vi "GEA2 Scale ERD Data.vi"(0 "HEWH ERD Data":T2 {"ERD Therm Data"."EEV Possition" format="%0.0f"; "ERD Therm Data"."T6" format="%.1f"; "ERD Therm Data"."T2" format="%.1f"; "ERD Therm Data"."T3a" format="%.1f"; "ERD Therm Data"."T3b" format="%.1f"; "ERD Therm Data"."T4" format="%.1f"; "ERD Therm Data"."T5" format="%.1f"; "ERD Therm Data"."Current" format="%.1f"}, 3 "Raw Data":string[](array[string]), 5 "ERD_Data_Bundled_Out":T5, 9 "Headers":string[](array[string]), 11 "Error In":errorcluster, 12 "LV Program":T1, 13 "Disable Electronic Mixing Valve (EMV) List":bool, 14 "Disable ERD (Main)":bool) -> (4 "ERD Array":string[][](array[string]), 15 "Error Out":errorcluster)   [LabVIEW 2016]
uses:
  type defs/HEWH ERD Data.ctl
  type defs/HEWH Faults.ctl
  type defs/HEWH Mixing Valve.ctl
  type defs/ERD_Data_Bundled.ctl
  Washer HCC/Washer HCC NEWFI/Washer Soft Load Box/type defs/ATC_Data.ctl
  Washer HCC/Washer HCC NEWFI/Washer Soft Load Box/type defs/Redundant.ctl
  Washer HCC/Washer HCC NEWFI/Washer Soft Load Box/type defs/Version.ctl
  Washer HCC/Washer HCC NEWFI/Washer Soft Load Box/type defs/Algorithms.ctl
  Washer HCC/Washer HCC NEWFI/Washer Soft Load Box/type defs/ERD_Always_Show.ctl
  Washer HCC/Washer HCC NEWFI/Washer Soft Load Box/type defs/Fault_Table_Info.ctl
  Save File/File Setup (Public)/Type Definition/Save File DOE LabView Program.ctl
  <vilib>/Utility/error.llb/whitespace.ctl
  Save File/File Setup.lvlib
panel:
  in  "Tab Control":enum32{"HEWH", "Washer"}(tab)
  # "Wet Load Size"
  # "Dry Load Size"
  # "OOB"
  # "Software Version"
  # "Critical Version"
  # "Non-Critical"
  # "XML Crit Ver"
  # "XML Non-Crit"
  # "Daily Build"
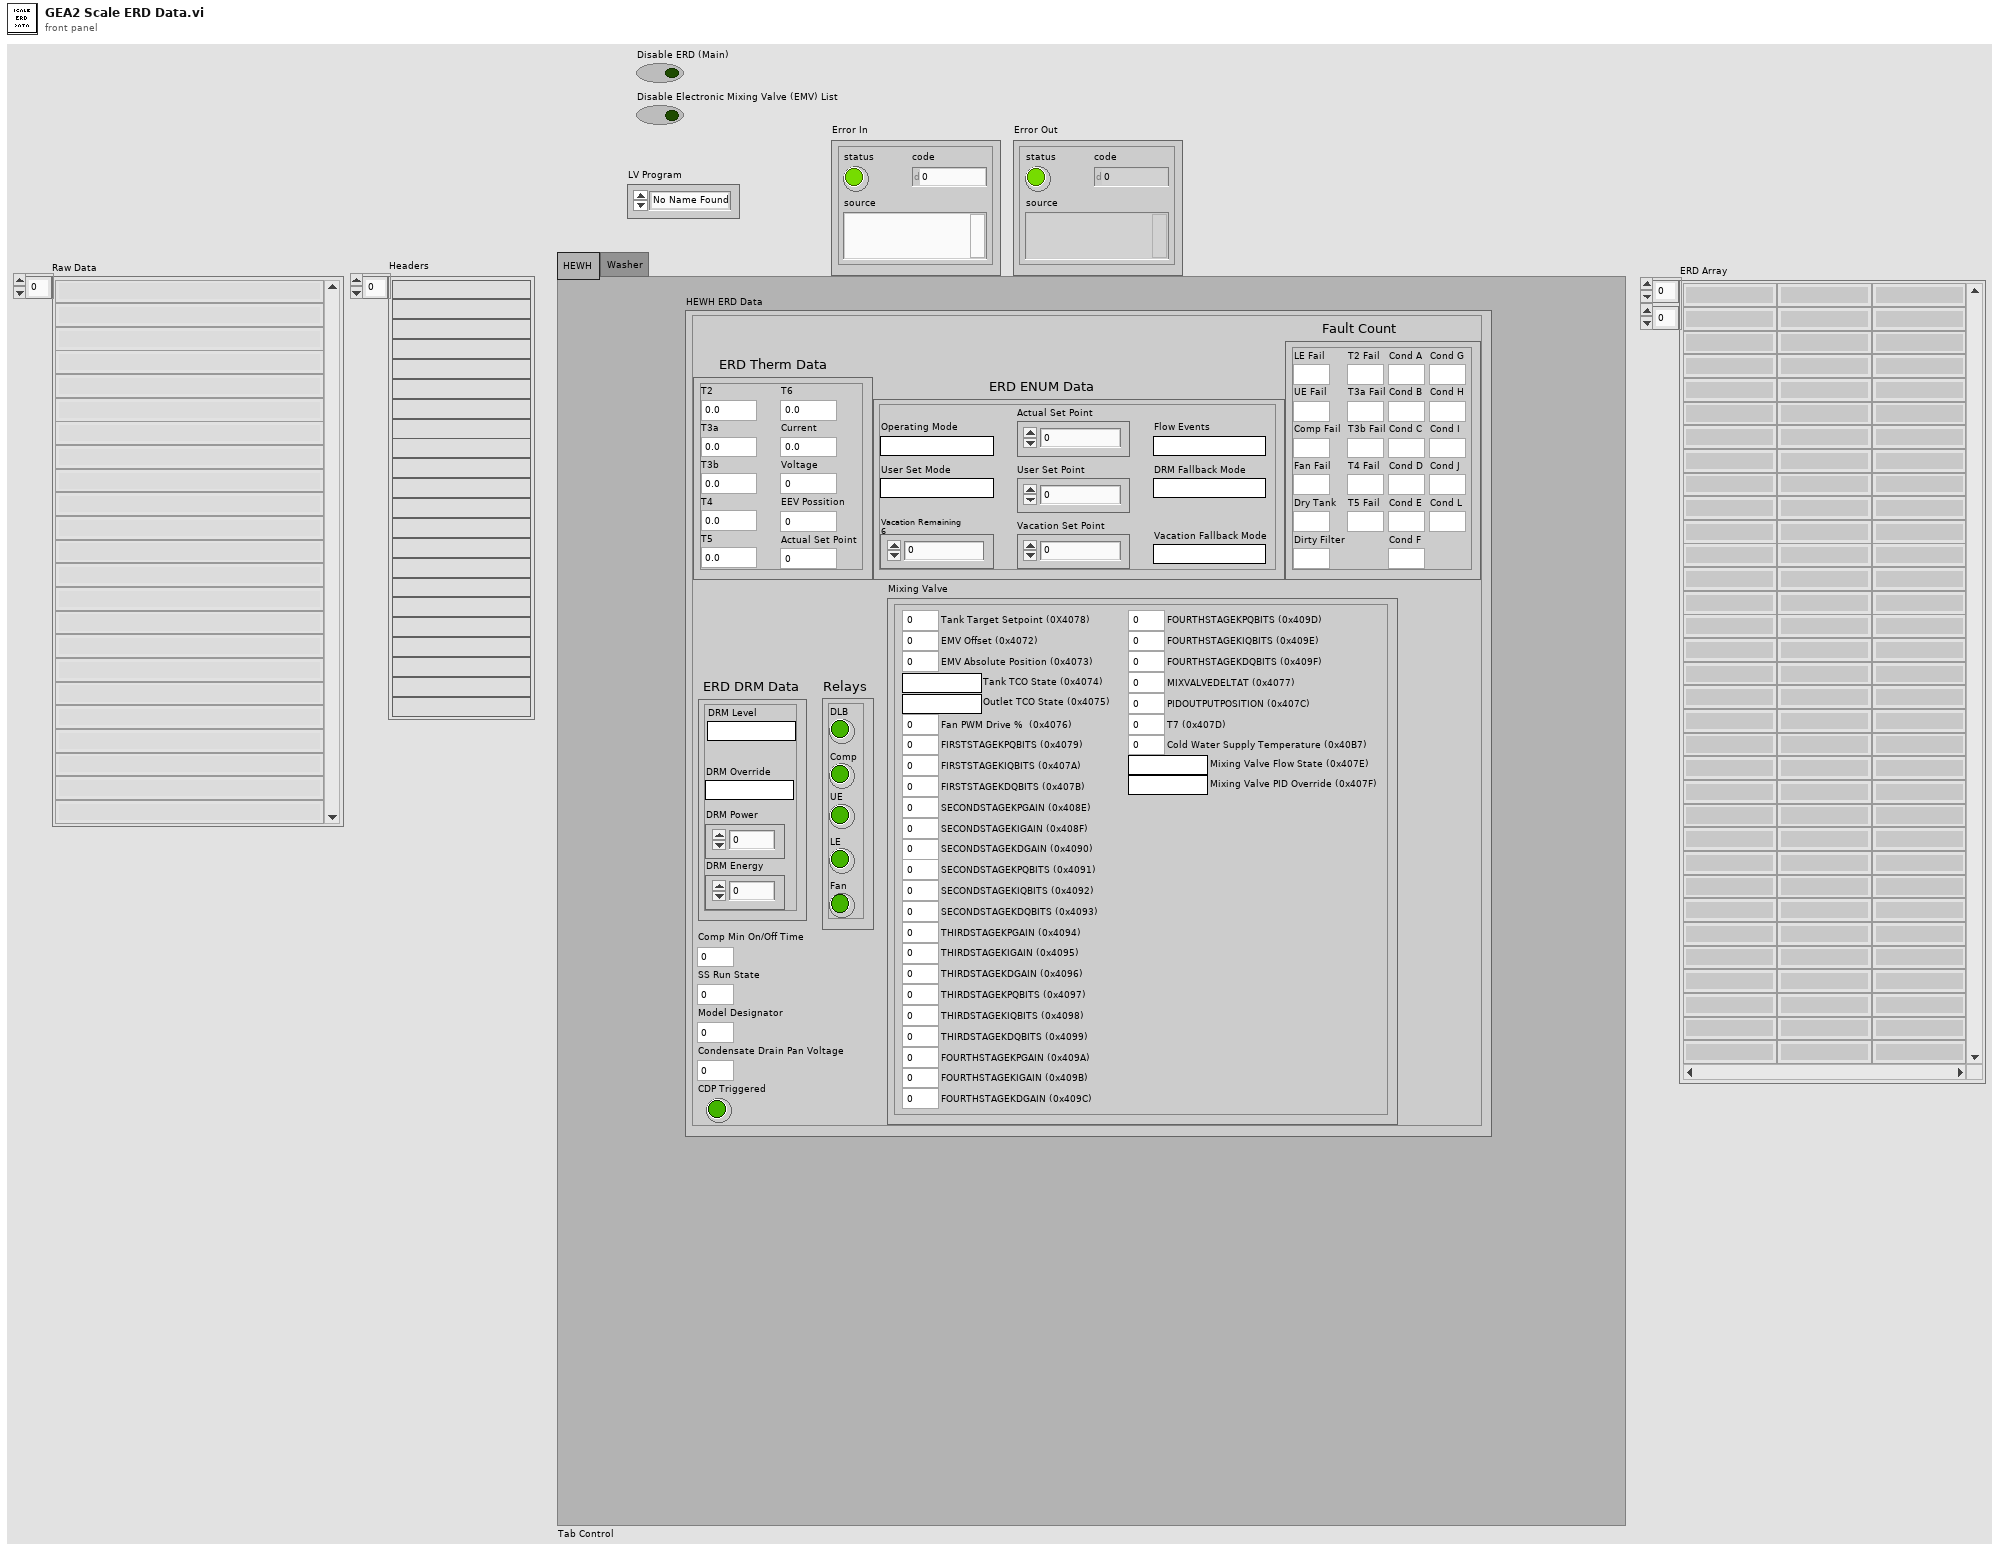
[diagram p1: front panel]
types:
  T1 = typedef "File Setup.lvlib/Save File DOE LabView Program.ctl" = enum16{"No Name Found", "DOE Stand", "Dishwasher Kitchen", "Portable Stand", "HEWH", "Dryer", "Dryer WILT", "HCC", "PRAT", "HEWH RLT", "Refrigeration"}
  T2 = typedef "HEWH ERD Data.ctl" = cluster{"ERD Therm Data":cluster{"T2":dbl, "T3a":dbl, "T3b":dbl, "T4":dbl, "T5":dbl, "T6":dbl, "Current":dbl, "Voltage":dbl, "EEV Possition":dbl, "Actual Set Point":dbl}, "ERD ENUM Data":cluster{"Actual Set Point":dbl, "Flow Events":string, "User Set Mode":string, "Operating Mode":string, "DRM Fallback Mode":string, "Vacation Fallback Mode":string, "User Set Point":dbl, "Vacation Set Point":dbl, "Vacation Remaining\n6":dbl}, "ERD DRM Data":cluster{"DRM Level":string, "DRM Override":string, "DRM Power":dbl, "DRM Energy":dbl}, "Fault Count":T3, "Relays":cluster{"DLB":bool, "Comp":bool, "UE":bool, "LE":bool, "Fan":bool}, "Comp Min On/Off Time":u16, "SS Run State":u16, "Condensate Drain Pan Voltage":u16, "CDP Triggered":bool, "Model Designator":u8, "Mixing Valve":T4}
  T3 = typedef "HEWH Faults.ctl" = cluster{"LE Fail":u32, "UE Fail":u32, "Comp Fail":u32, "T2 Fail":u32, "T3a Fail":u32, "T3b Fail":u32, "T4 Fail":u32, "T5 Fail":u32, "Cond A":u32, "Cond B":u32, "Cond C":u32, "Cond D":u32, "Cond E":u32, "Cond F":u32, "Cond G":u32, "Cond H":u32, "Cond I":u32, "Cond J":u32, "Cond L":u32, "Fan Fail":u32, "Dirty Filter":u32, "Dry Tank":u32}
  T4 = typedef "HEWH Mixing Valve.ctl" = cluster{"Tank Target Setpoint (0X4078)":dbl, "EMV Offset (0x4072)":dbl, "EMV Absolute Position (0x4073)":dbl, "Tank TCO State (0x4074)":string, "Outlet TCO State (0x4075)":string, "Fan PWM Drive %  (0x4076)":dbl, "FIRSTSTAGEKPQBITS (0x4079)":dbl, "FIRSTSTAGEKIQBITS (0x407A)":dbl, "FIRSTSTAGEKDQBITS (0x407B)":dbl, "SECONDSTAGEKPGAIN (0x408E)":dbl, "SECONDSTAGEKIGAIN (0x408F)":dbl, "SECONDSTAGEKDGAIN (0x4090)":dbl, "SECONDSTAGEKPQBITS (0x4091)":dbl, "SECONDSTAGEKIQBITS (0x4092)":dbl, "SECONDSTAGEKDQBITS (0x4093)":dbl, "THIRDSTAGEKPGAIN (0x4094)":dbl, "THIRDSTAGEKIGAIN (0x4095)":dbl, "THIRDSTAGEKDGAIN (0x4096)":dbl, "THIRDSTAGEKPQBITS (0x4097)":dbl, "THIRDSTAGEKIQBITS (0x4098)":dbl, "THIRDSTAGEKDQBITS (0x4099)":dbl, "FOURTHSTAGEKPGAIN (0x409A)":dbl, "FOURTHSTAGEKIGAIN (0x409B)":dbl, "FOURTHSTAGEKDGAIN (0x409C)":dbl, "FOURTHSTAGEKPQBITS (0x409D)":dbl, "FOURTHSTAGEKIQBITS (0x409E)":dbl, "FOURTHSTAGEKDQBITS (0x409F)":dbl, "MIXVALVEDELTAT (0x4077)":dbl, "PIDOUTPUTPOSITION (0x407C)":dbl, "T7 (0x407D)":dbl, "Cold Water Supply Temperature (0x40B7)":dbl, "Mixing Valve Flow State (0x407E)":string, "Mixing Valve PID Override (0x407F)":string}
  T5 = typedef "ERD_Data_Bundled.ctl" = cluster{"ATC Data":T6, "Redundant Micro":T7, "Version":T8, "Algorithm Data":T9, "ERD_Always Show":T10, "ERD Graph  Ind":cluster{"ERD Value 1":dbl, "ERD Value 2":dbl, "ERD Value 3":dbl}, "Personality Set":u8, "Fault Table Entry":T11[]}
  T6 = typedef "ATC_Data.ctl" = cluster{"Current Tub Gallons":dbl, "Hot Gallons":dbl, "Cold Gallons":dbl, "Target Gallons":dbl, "Current Water Temp":dbl, "Target Level":u32, "Target Bath Temp":dbl, "Current Bath Temp ":dbl, "Cold Inlet Temp":dbl, "Hot Inlet Temp":dbl, "Warm Inlet Temp":dbl, "Hot Seg Valve Time":u16, "Cold Seg Valve Time ":u16, "User Temp Level":string, "Segment Gallons":dbl}
  T7 = typedef "Redundant.ctl" = cluster{"Version":string, "Personality":u8, "Pressure ":dbl, "Shaft Speed":u16, "Modeshift Feedback":string, "Lid Switch":bool, "Lid Lock":bool, "Triac Enable":bool, "Drain Pump":bool, "Lid Lock Motor Speed Safety Interlock":bool, "Flood Condition State":bool, "Lid Open Fault State":bool, "Access To Moving Parts State":bool, "Heartbeat":bool, "Motor Enable":bool, "Lid Unlock Fault State":bool}
  T8 = typedef "Version.ctl" = cluster{"Critical Major":string, "Critical Minor":string, "Non-Critical Minor":string, "Non-Critical Major":string, "XML Crit Minor":string, "XMLCrit Major":string, "Daily Rev":string, "XML Non-crit Minor":string, "Xml Non-crit Major":string}
  T9 = typedef "Algorithms.ctl" = cluster{"Wet Load Gal":dbl, "Target Gallons":dbl, "Load Type":string, "Load Size":string, "Coast Time":u16, "Ramp Time":u16, "Ramp  Speed":u16, "Ramp Avg Current":dbl, "OOB Redist Req":bool, "OOB Detected in S-S":bool, "Max Accel in Accel":i32, "Max Jerk in Accel":i32, "Max Jerk in S-S":i32, "OOB Detected in Accel":bool, "Partial Coast Time":u16, "Dry Load Size":dbl, "Ramp Line Voltage ":dbl, "Coast Line Voltage":dbl}
  T10 = typedef "ERD_Always_Show.ctl" = cluster{"Basket Speed (RPM)":u16, "Machine State":string, "Tub Volume (Gal)":dbl, "Pressure (inches H20)":dbl, "Lid Switch ":bool, "Current RMS (Amps)":dbl, "Cycle Selected":string, "Lid Lock Status":string, "Mode Shift Status":string, "Spray/Rinse Valve":bool, "Fabric Soft Valve":bool, "Drain Pump":bool, "Recirc. Pump":bool, "Cycle Engine State":string, "Hot  Water Valve":bool, "Cold Water Valve":bool, "Motor Profile":string, "Motor Profile Status":string, "Motor Mode":string, "ME Relay":bool, "Cycle Count":u32, "Deep Rinse / FS":bool, "My Cycle":bool, "Soil Level":string, "Spin Level":string, "Stain":string, "Temp Level":string, "Load Size":string, "Delay Time":u16, "Soak Time":u16, "Deep Fill":bool, "Warm Rinse":bool, "Auto Soak Level":string, "Extra Rinse":bool, "Wet Load Gallons":dbl, "Target Gallons":dbl, "Sub-Cycle":string, "Load Type":string, "Target Level (inches)":u32, "Valve Relay":bool, "Dry Load Size":dbl, "Shaft Speed (RPM) ":u16, "MS Motor":bool, "Mode Shift FB":bool, "Target Bath Temp (F)":dbl, "Temperature (F)":dbl, "Current Bath Temp (F)":dbl, "Lid Lock FB":string, "Lid Lock Req State":string, "Remaining Cycle Time (s)":dbl, "Available Free Stack %":u8, "Child Safety":bool, "Target Speed (RPM)":u16, "Reset Source":string}
  T11 = typedef "Fault_Table_Info.ctl" = cluster{"Cycle Count":u32, " Runtime (min) ":u32, "Fault Status":string, "Fault ID":string, "Fault Count":u16}
  T12 = typedef "whitespace.ctl" = u16
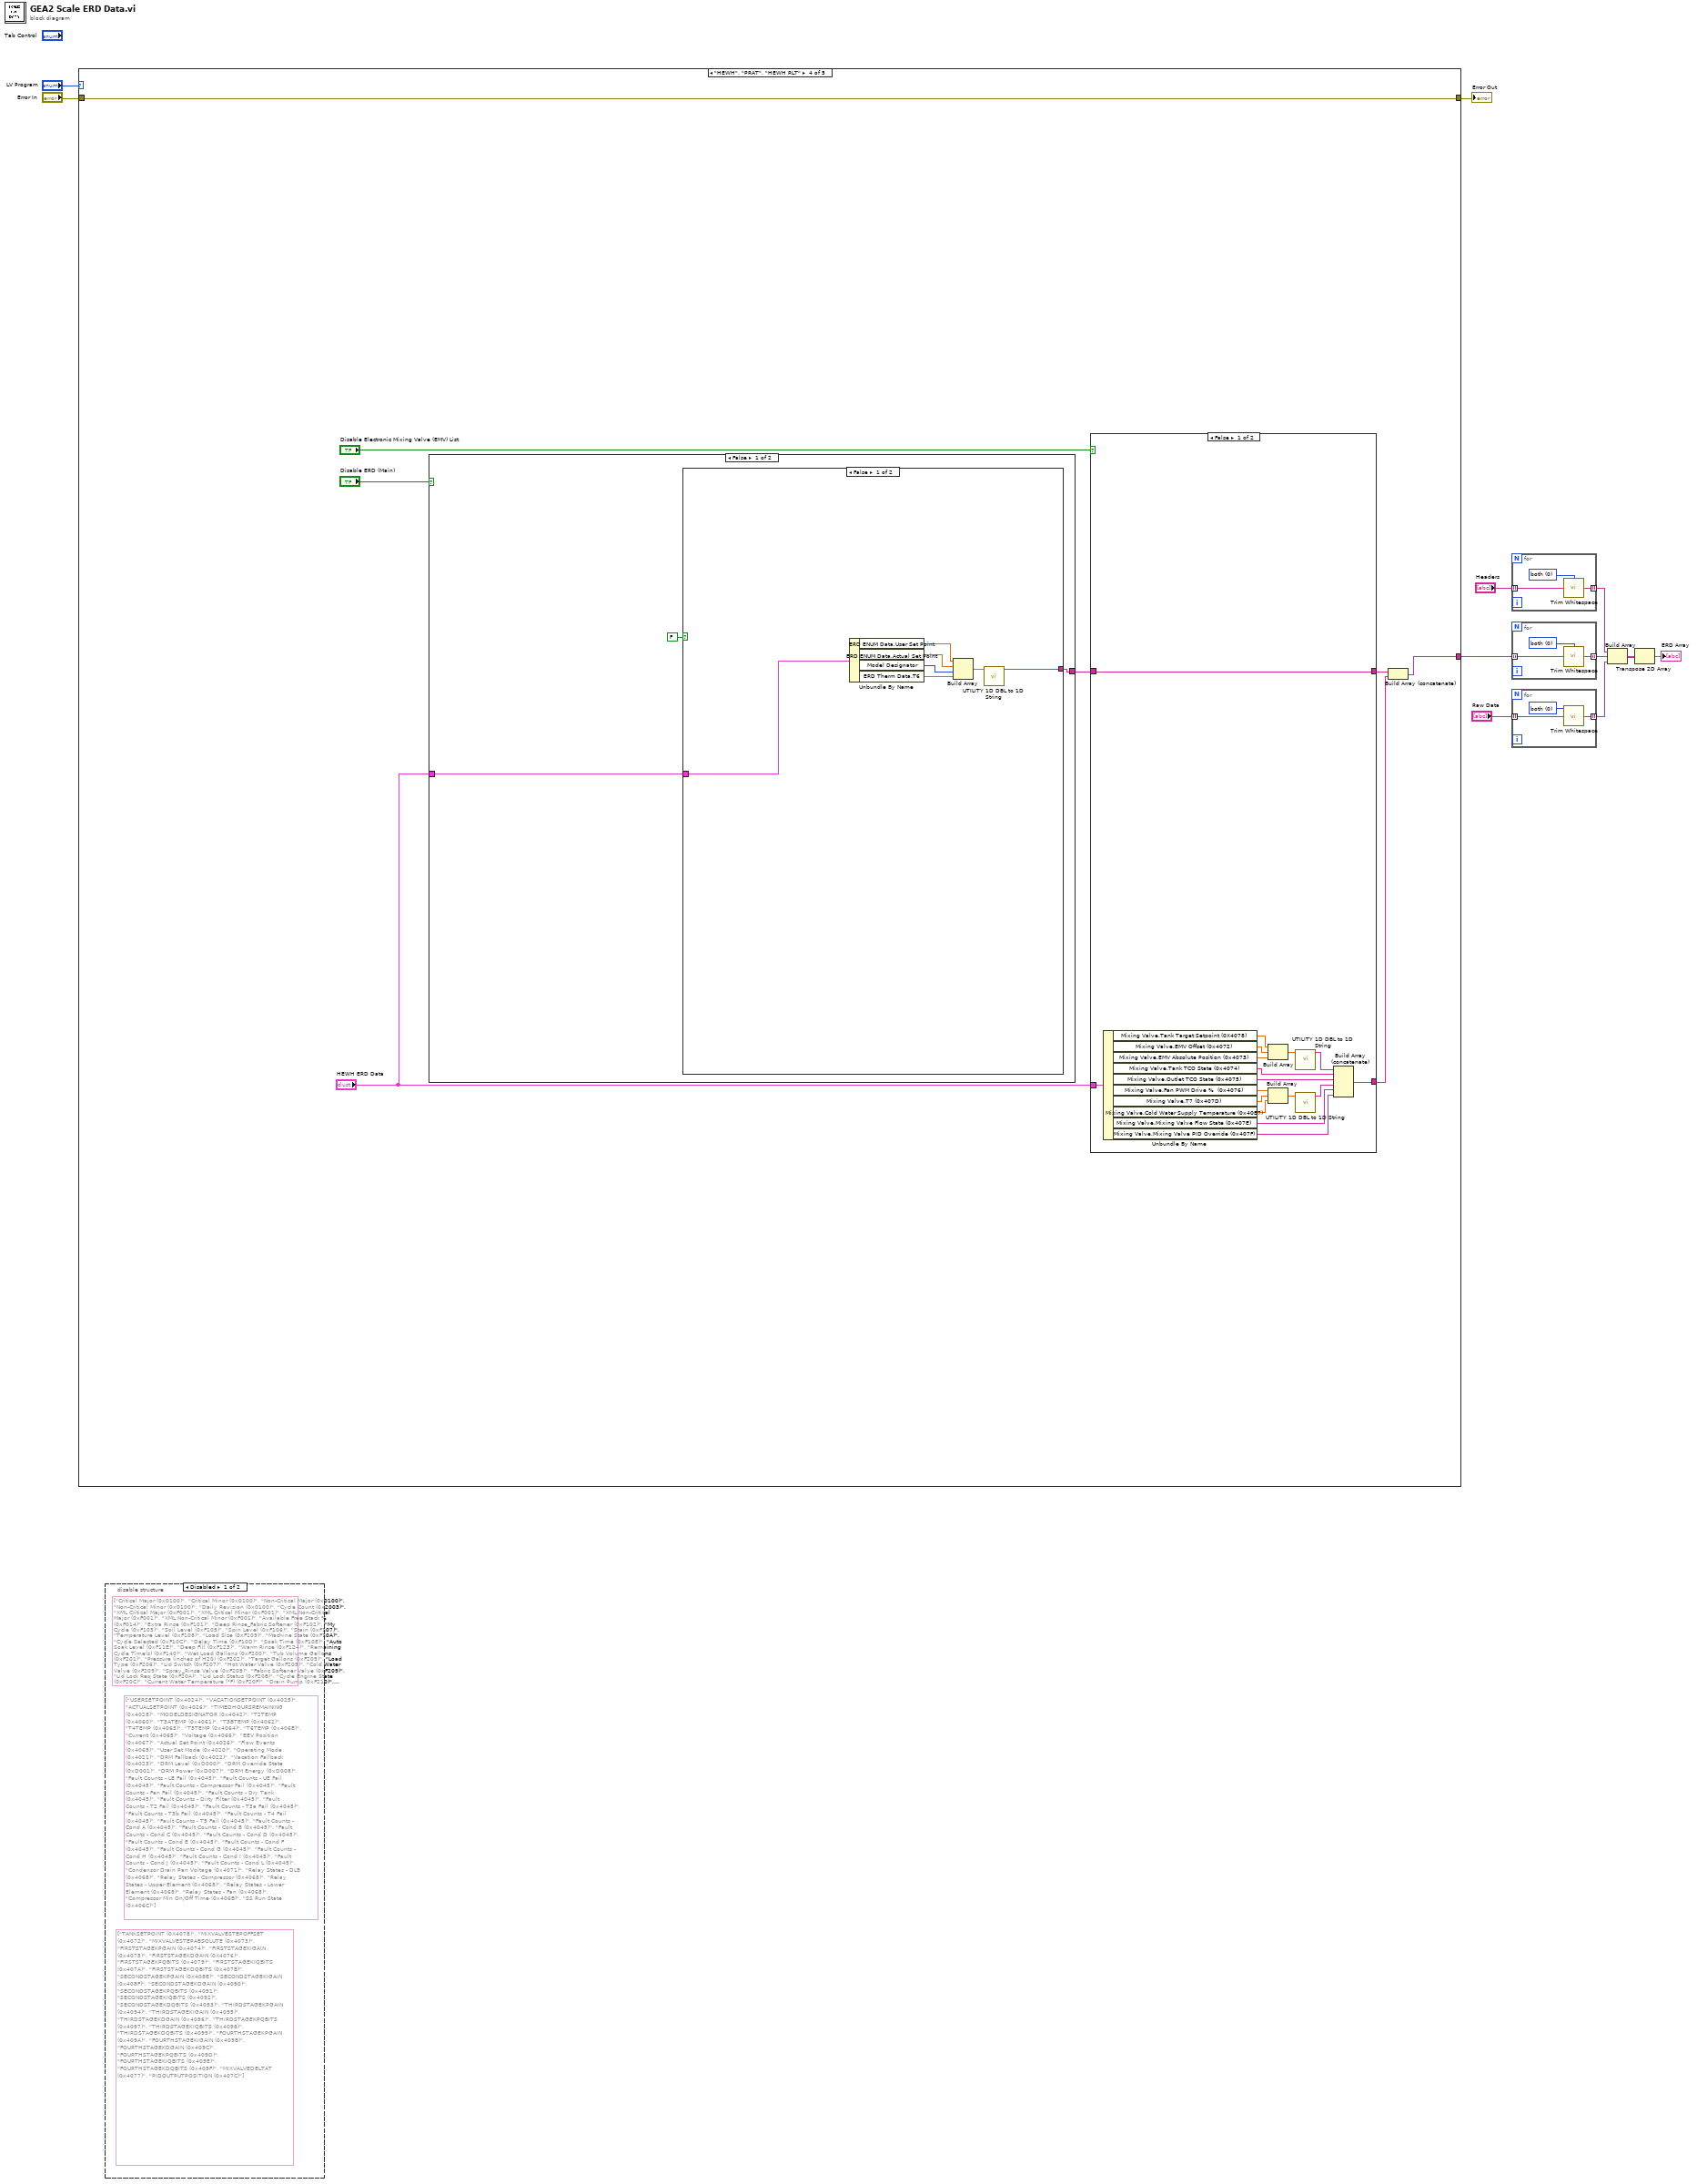
[diagram p0: block diagram]
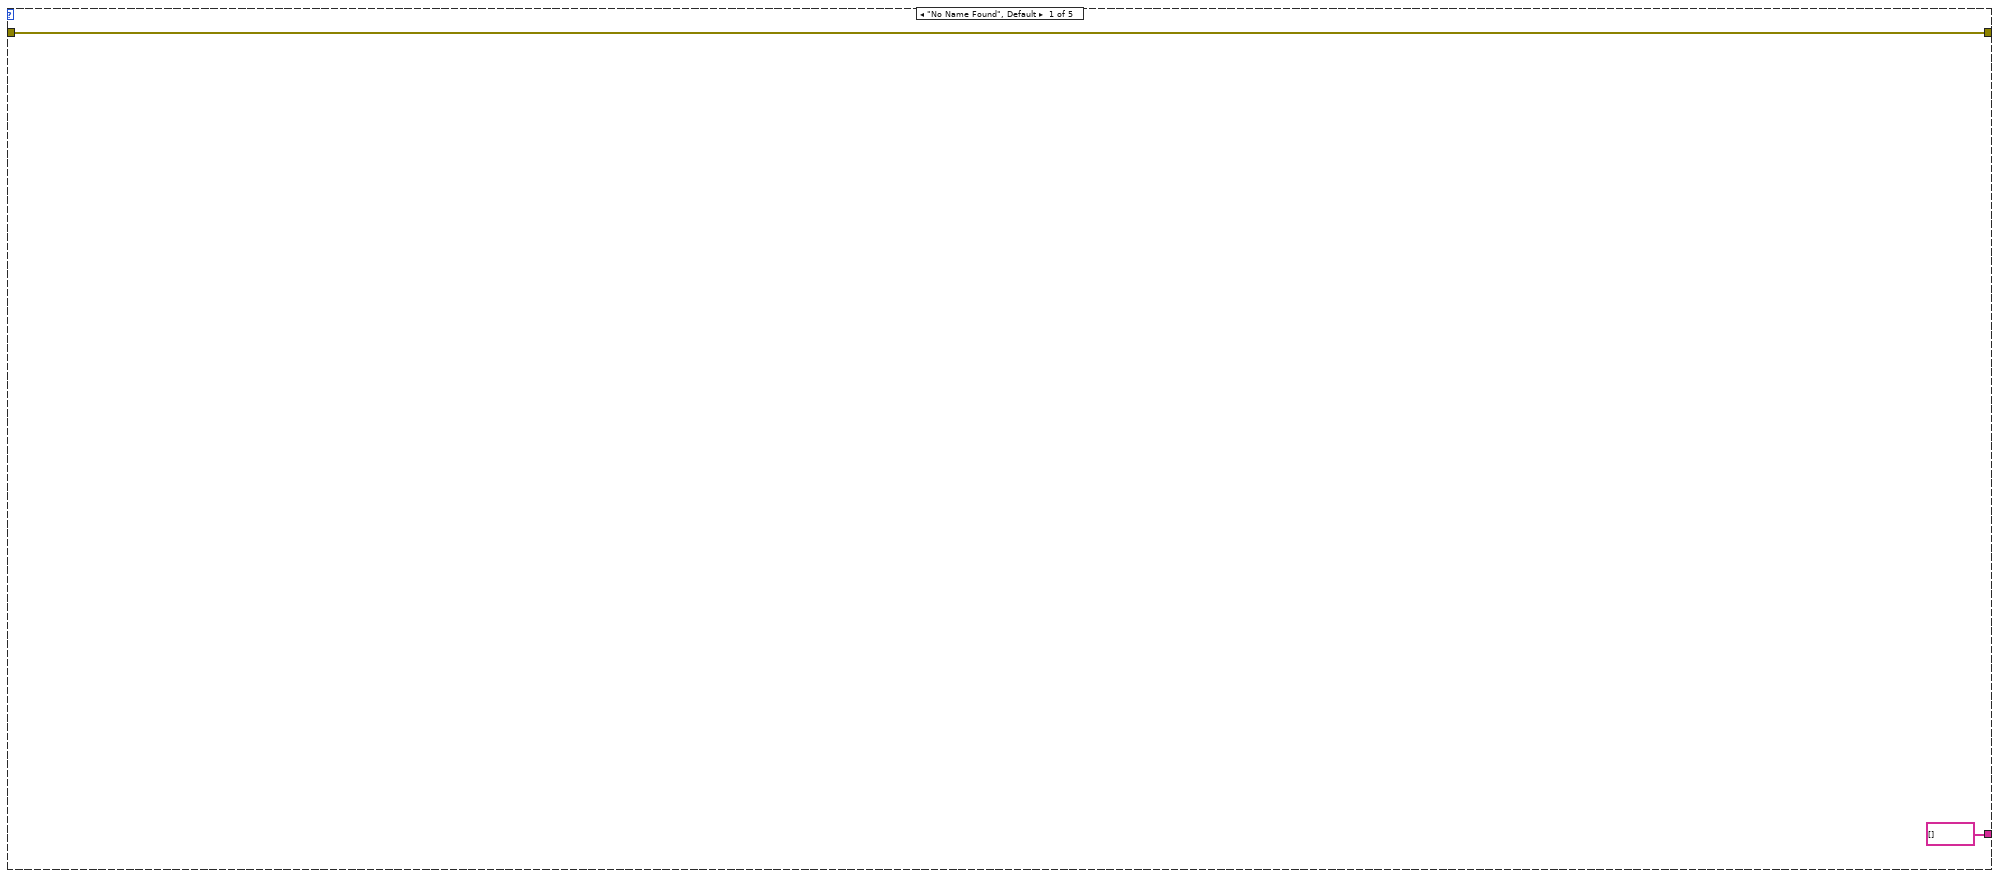
[diagram p3: hidden frame]
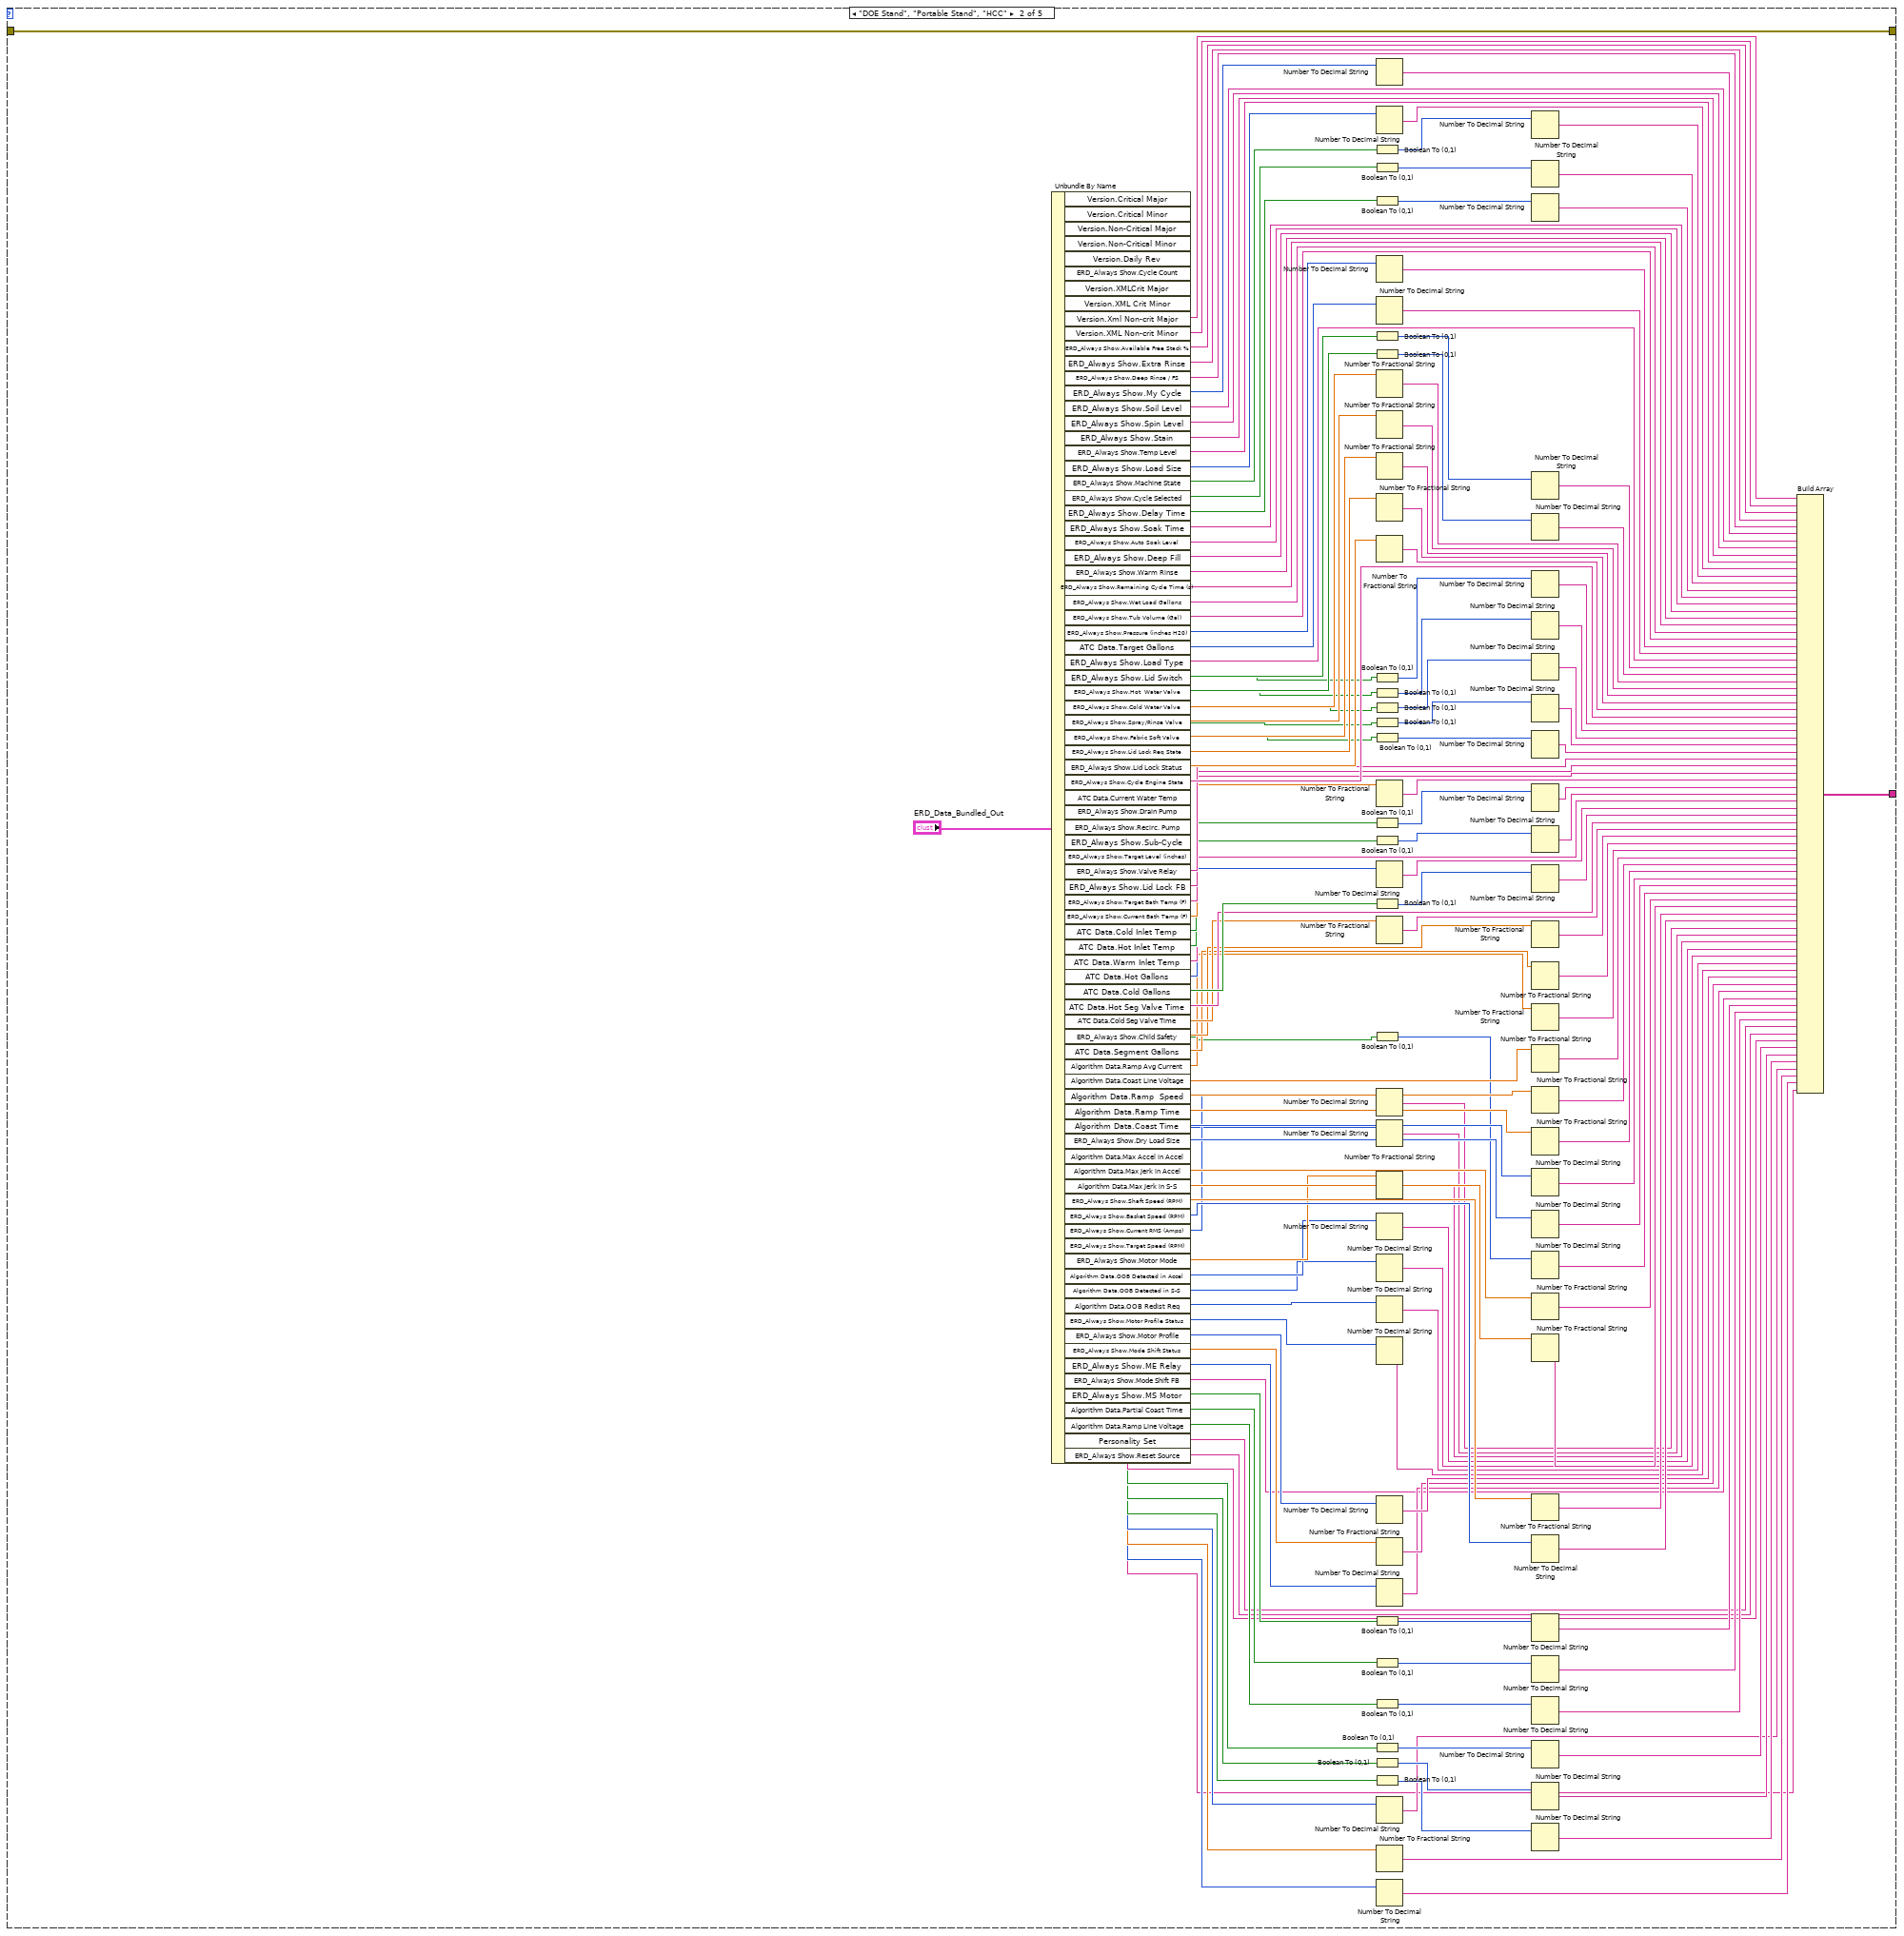
[diagram p4: hidden frame]
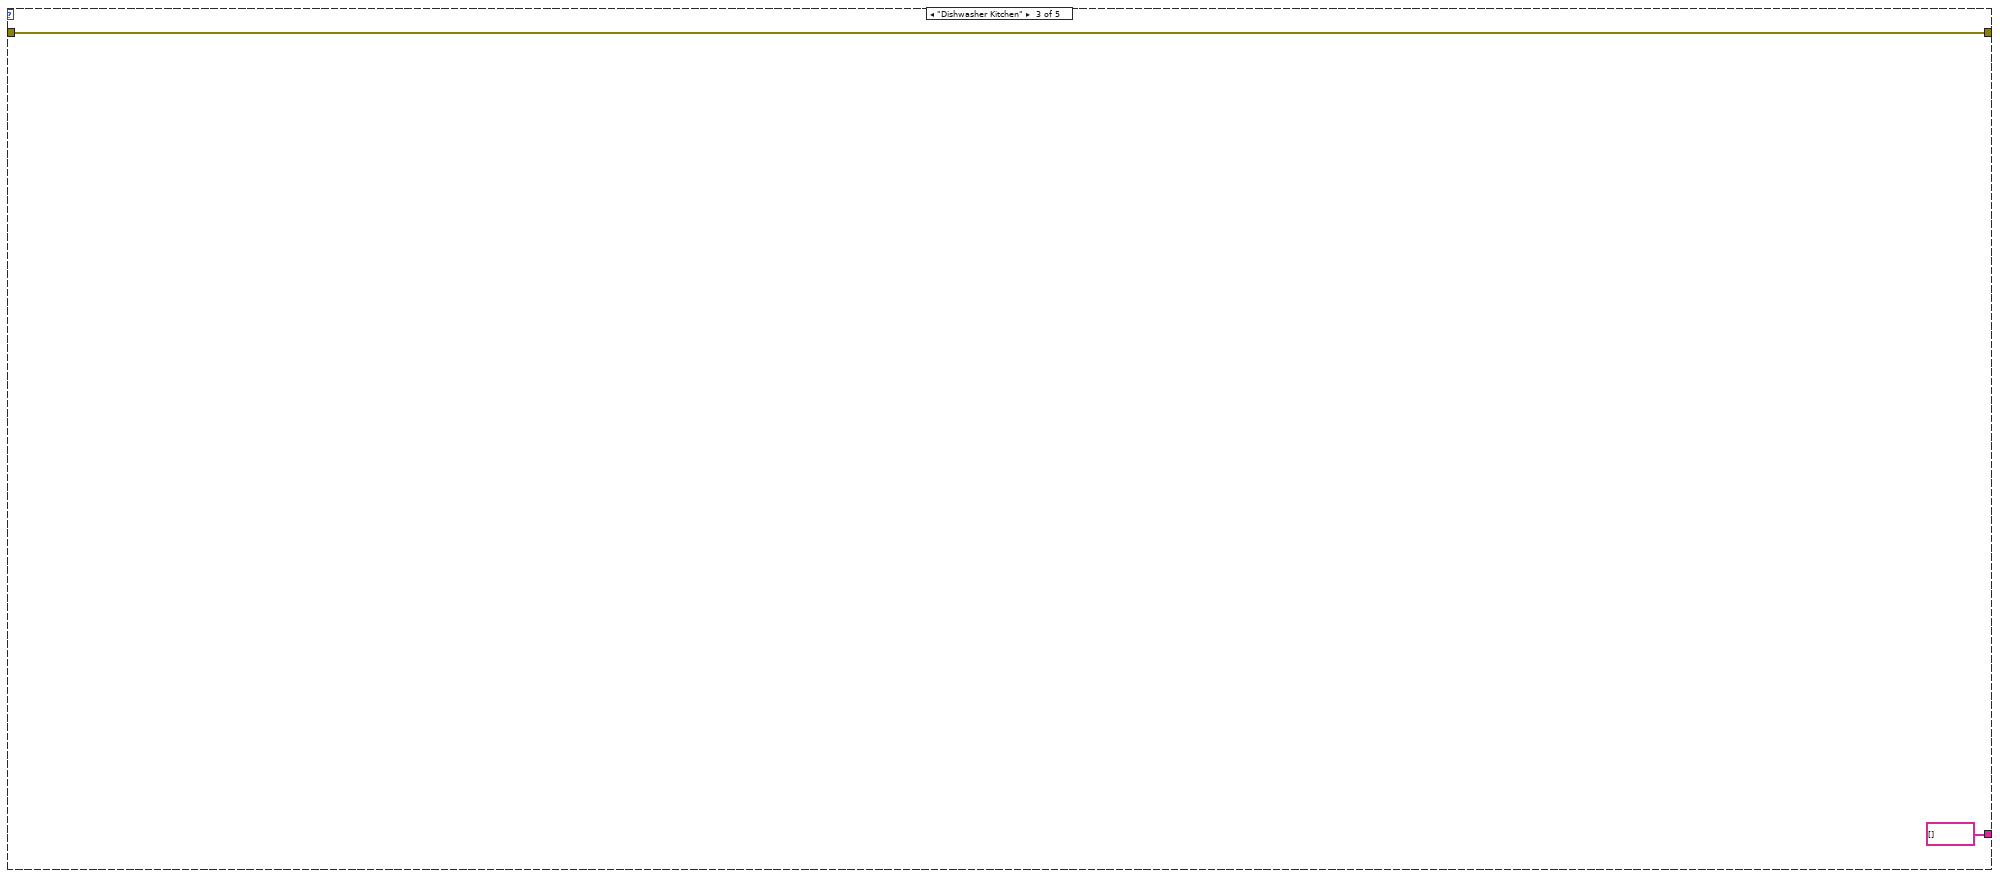
[diagram p5: hidden frame]
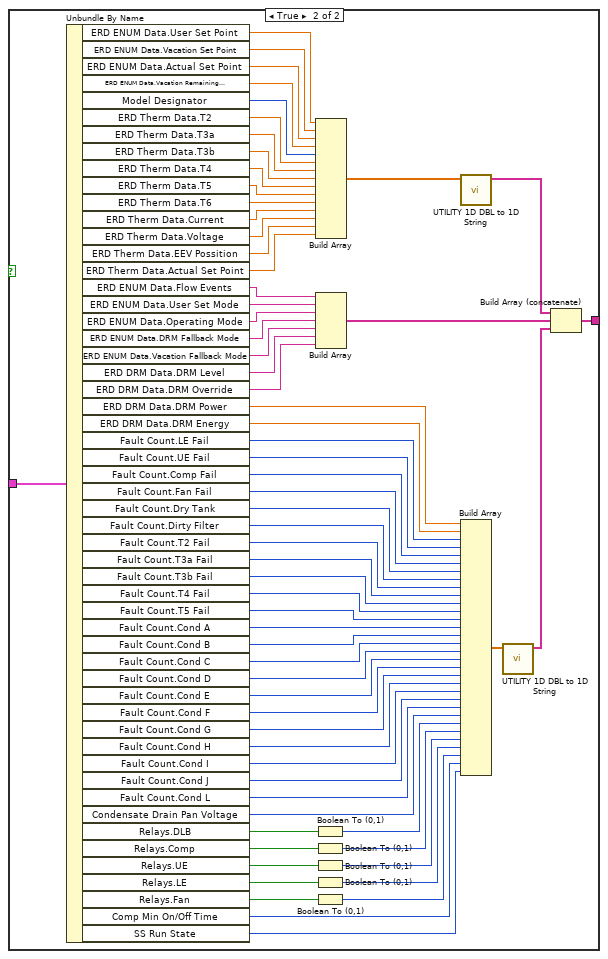
[diagram p6: hidden frame]
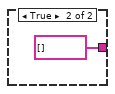
[diagram p7: hidden frame]
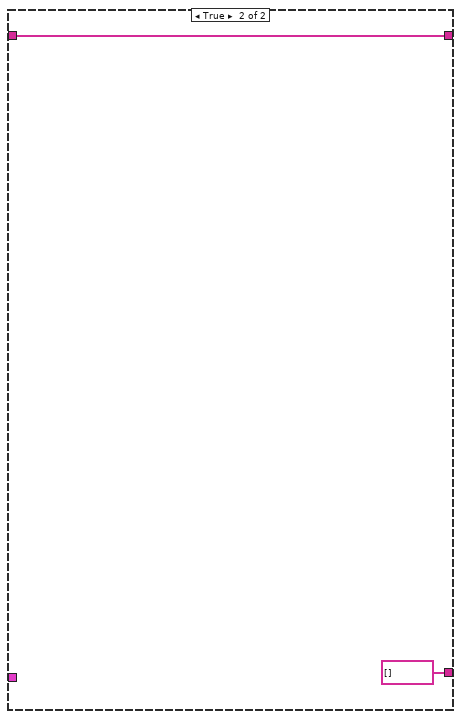
[diagram p8: hidden frame]
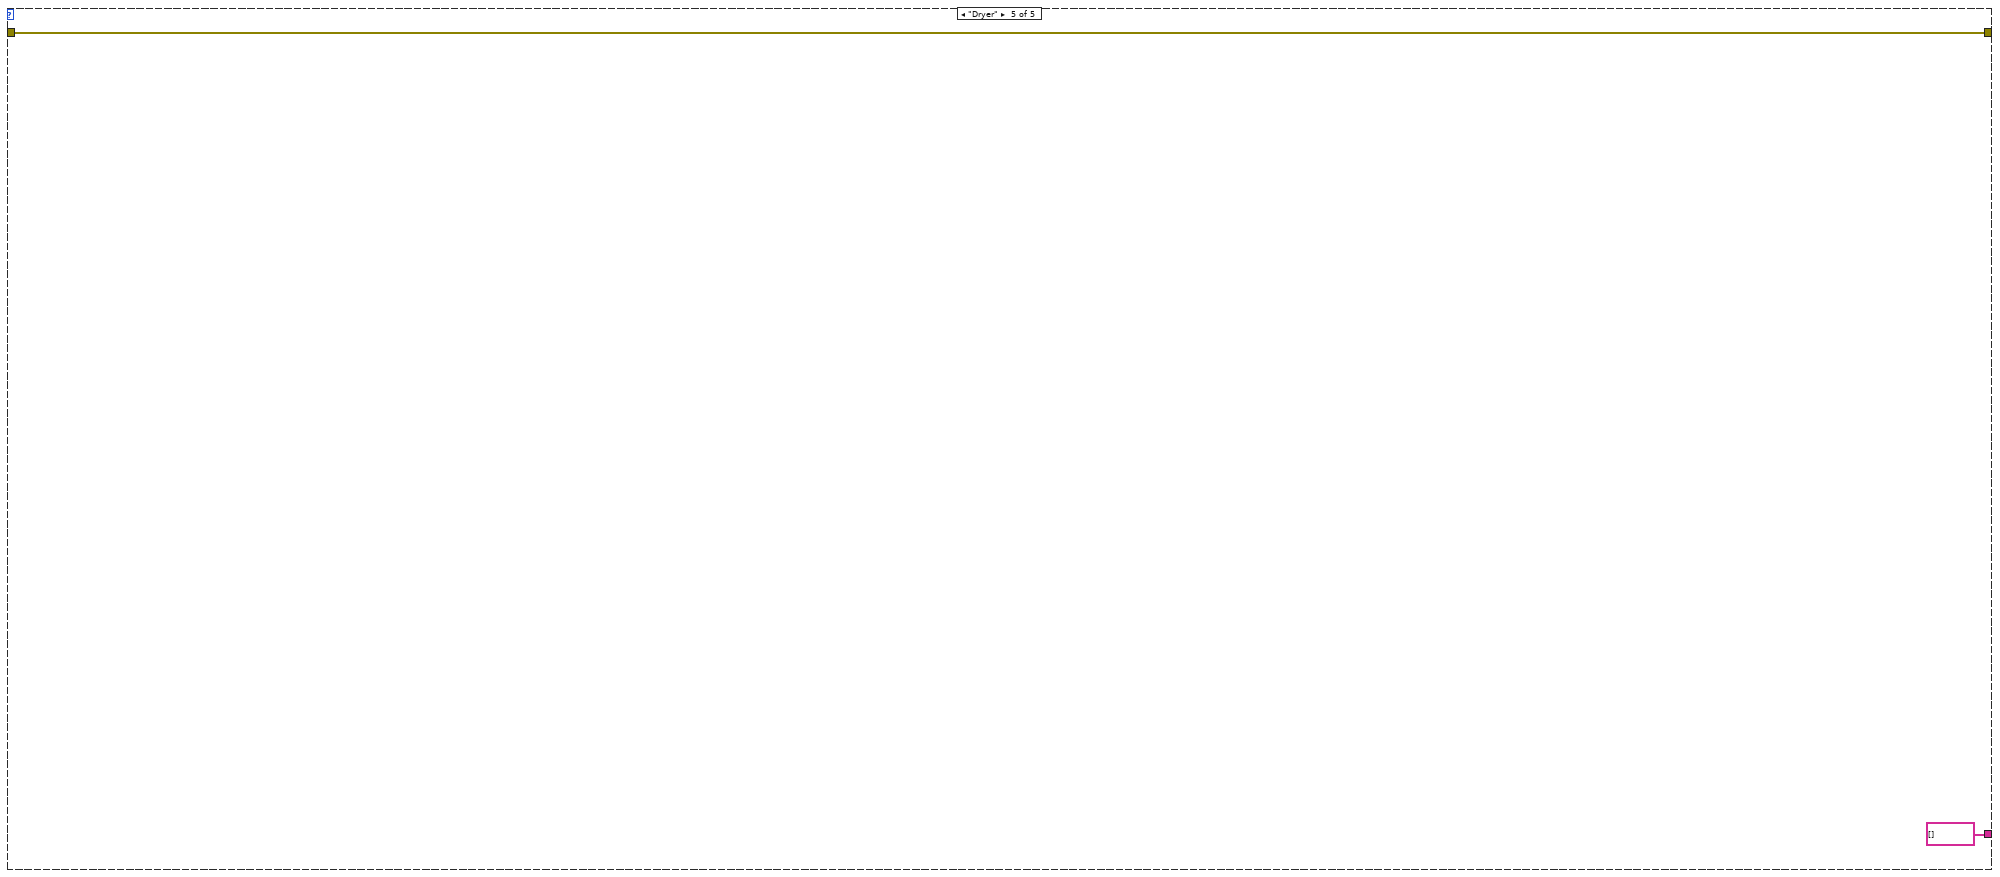
[diagram p9: hidden frame]
diagram:
  n1 = case shown="\"HEWH\", \"PRAT\", \"HEWH RLT\"" "LV Program" {
    tunnel: "Error In" -> [w13 w178 w180 w188 w286]
    tunnel: [w13 w178 w180 w188 w286] -> w7
    tunnel: [string[] [] ("1D String") w14 string[] [] ("1D String") w182 string[] [] ("1D String")] -> w2
    frame "No Name Found", Default {
    }
    frame "DOE Stand", "Portable Stand", "HCC" {
      n2 = Unbundle By Name("ERD_Data_Bundled_Out") -> ("Version.Critical Major"=w176:string, "Version.Critical Minor"=w175:string, "Version.Non-Critical Major"=w174:string, "Version.Non-Critical Minor"=w173:string, "Version.Daily Rev"=w172:string, "ERD_Always Show.Cycle Count"=w171:u32, "Version.XMLCrit Major"=w169:string, "Version.XML Crit Minor"=w168:string, "Version.Xml Non-crit Major"=w167:string, "Version.XML Non-crit Minor"=w166:string, "ERD_Always Show.Available Free Stack %"=w165:u8, "ERD_Always Show.Extra Rinse"=w163:bool, "ERD_Always Show.Deep Rinse / FS"=w159:bool, "ERD_Always Show.My Cycle"=w156:bool, "ERD_Always Show.Soil Level"=w154:string, "ERD_Always Show.Spin Level"=w153:string, "ERD_Always Show.Stain"=w152:string, "ERD_Always Show.Temp Level"=w151:string, "ERD_Always Show.Load Size"=w150:string, "ERD_Always Show.Machine State"=w149:string, "ERD_Always Show.Cycle Selected"=w148:string, "ERD_Always Show.Delay Time"=w147:u16, "ERD_Always Show.Soak Time"=w145:u16, "ERD_Always Show.Auto Soak Level"=w143:string, "ERD_Always Show.Deep Fill"=w141:bool, "ERD_Always Show.Warm Rinse"=w138:bool, "ERD_Always Show.Remaining Cycle Time (s)"=w136:dbl, "ERD_Always Show.Wet Load Gallons"=w134:dbl, "ERD_Always Show.Tub Volume (Gal)"=w132:dbl, "ERD_Always Show.Pressure (inches H20)"=w130:dbl, "ATC Data.Target Gallons"=w128:dbl, "ERD_Always Show.Load Type"=w126:string, "ERD_Always Show.Lid Switch"=w124:bool, "ERD_Always Show.Hot  Water Valve"=w121:bool, "ERD_Always Show.Cold Water Valve"=w118:bool, "ERD_Always Show.Spray/Rinse Valve"=w115:bool, "ERD_Always Show.Fabric Soft Valve"=w112:bool, "ERD_Always Show.Lid Lock Req State"=w110:string, "ERD_Always Show.Lid Lock Status"=w109:string, "ERD_Always Show.Cycle Engine State"=w108:string, "ATC Data.Current Water Temp"=w107:dbl, "ERD_Always Show.Drain Pump"=w104:bool, "ERD_Always Show.Recirc. Pump"=w101:bool, "ERD_Always Show.Sub-Cycle"=w99:string, "ERD_Always Show.Target Level (inches)"=w98:u32, "ERD_Always Show.Valve Relay"=w95:bool, "ERD_Always Show.Lid Lock FB"=w93:string, "ERD_Always Show.Target Bath Temp (F)"=w92:dbl, "ERD_Always Show.Current Bath Temp (F)"=w90:dbl, "ATC Data.Cold Inlet Temp"=w88:dbl, "ATC Data.Hot Inlet Temp"=w86:dbl, "ATC Data.Warm Inlet Temp"=w84:dbl, "ATC Data.Hot Gallons"=w82:dbl, "ATC Data.Cold Gallons"=w80:dbl, "ATC Data.Hot Seg Valve Time"=w78:u16, "ATC Data.Cold Seg Valve Time"=w76:u16, "ERD_Always Show.Child Safety"=w73:bool, "ATC Data.Segment Gallons"=w71:dbl, "Algorithm Data.Ramp Avg Current"=w69:dbl, "Algorithm Data.Coast Line Voltage"=w67:dbl, "Algorithm Data.Ramp  Speed"=w65:u16, "Algorithm Data.Ramp Time"=w63:u16, "Algorithm Data.Coast Time"=w61:u16, "ERD_Always Show.Dry Load Size"=w59:dbl, "Algorithm Data.Max Accel in Accel"=w57:i32, "Algorithm Data.Max Jerk in Accel"=w55:i32, "Algorithm Data.Max Jerk in S-S"=w53:i32, "ERD_Always Show.Shaft Speed (RPM)"=w51:u16, "ERD_Always Show.Basket Speed (RPM)"=w49:u16, "ERD_Always Show.Current RMS (Amps)"=w47:dbl, "ERD_Always Show.Target Speed (RPM)"=w45:u16, "ERD_Always Show.Motor Mode"=w43:string, "Algorithm Data.OOB Detected in Accel"=w41:bool, "Algorithm Data.OOB Detected in S-S"=w38:bool, "Algorithm Data.OOB Redist Req"=w35:bool, "ERD_Always Show.Motor Profile Status"=w33:string, "ERD_Always Show.Motor Profile"=w32:string, "ERD_Always Show.Mode Shift Status"=w31:string, "ERD_Always Show.ME Relay"=w29:bool, "ERD_Always Show.Mode Shift FB"=w26:bool, "ERD_Always Show.MS Motor"=w23:bool, "Algorithm Data.Partial Coast Time"=w21:u16, "Algorithm Data.Ramp Line Voltage"=w19:dbl, "Personality Set"=w17:u8, "ERD_Always Show.Reset Source"=w15:string)
      n3 = Boolean To (0,1)(Boolean=w163) -> (0, 1=w162:i16)
      n4 = Boolean To (0,1)(Boolean=w159) -> (0, 1=w160:i16)
      n5 = Boolean To (0,1)(Boolean=w156) -> (0, 1=w157:i16)
      n6 = Boolean To (0,1)(Boolean=w141) -> (0, 1=w142:i16)
      n7 = Boolean To (0,1)(Boolean=w138) -> (0, 1=w139:i16)
      n8 = Boolean To (0,1)(Boolean=w124) -> (0, 1=w125:i16)
      n9 = Boolean To (0,1)(Boolean=w121) -> (0, 1=w122:i16)
      n10 = Boolean To (0,1)(Boolean=w118) -> (0, 1=w119:i16)
      n11 = Boolean To (0,1)(Boolean=w115) -> (0, 1=w116:i16)
      n12 = Boolean To (0,1)(Boolean=w112) -> (0, 1=w113:i16)
      n13 = Boolean To (0,1)(Boolean=w104) -> (0, 1=w105:i16)
      n14 = Boolean To (0,1)(Boolean=w101) -> (0, 1=w102:i16)
      n15 = Boolean To (0,1)(Boolean=w95) -> (0, 1=w96:i16)
      n16 = Boolean To (0,1)(Boolean=w73) -> (0, 1=w74:i16)
      n17 = Boolean To (0,1)(Boolean=w41) -> (0, 1=w42:i16)
      n18 = Boolean To (0,1)(Boolean=w38) -> (0, 1=w39:i16)
      n19 = Boolean To (0,1)(Boolean=w35) -> (0, 1=w36:i16)
      n20 = Boolean To (0,1)(Boolean=w29) -> (0, 1=w30:i16)
      n21 = Boolean To (0,1)(Boolean=w26) -> (0, 1=w27:i16)
      n22 = Boolean To (0,1)(Boolean=w23) -> (0, 1=w24:i16)
      n23 = Number To Decimal String(number=w171) -> (decimal integer string=w170:string)  [unwired: 1 in]
      n24 = Number To Decimal String(number=w165) -> (decimal integer string=w164:string)  [unwired: 1 in]
      n25 = Number To Decimal String(number=w147) -> (decimal integer string=w146:string)  [unwired: 1 in]
      n26 = Number To Decimal String(number=w145) -> (decimal integer string=w144:string)  [unwired: 1 in]
      n27 = Number To Fractional String(number=w136) -> (F-format string=w135:string)  [unwired: 3 in]
      n28 = Number To Fractional String(number=w134) -> (F-format string=w133:string)  [unwired: 3 in]
      n29 = Number To Fractional String(number=w132) -> (F-format string=w131:string)  [unwired: 3 in]
      n30 = Number To Fractional String(number=w130) -> (F-format string=w129:string)  [unwired: 3 in]
      n31 = Number To Fractional String(number=w128) -> (F-format string=w127:string)  [unwired: 3 in]
      n32 = Number To Fractional String(number=w107) -> (F-format string=w106:string)  [unwired: 3 in]
      n33 = Number To Decimal String(number=w98) -> (decimal integer string=w97:string)  [unwired: 1 in]
      n34 = Number To Fractional String(number=w92) -> (F-format string=w91:string)  [unwired: 3 in]
      n35 = Number To Decimal String(number=w63) -> (decimal integer string=w62:string)  [unwired: 1 in]
      n36 = Number To Decimal String(number=w61) -> (decimal integer string=w60:string)  [unwired: 1 in]
      n37 = Number To Fractional String(number=w59) -> (F-format string=w58:string)  [unwired: 3 in]
      n38 = Number To Decimal String(number=w57) -> (decimal integer string=w56:string)  [unwired: 1 in]
      n39 = Number To Decimal String(number=w55) -> (decimal integer string=w54:string)  [unwired: 1 in]
      n40 = Number To Decimal String(number=w53) -> (decimal integer string=w52:string)  [unwired: 1 in]
      n41 = Number To Decimal String(number=w51) -> (decimal integer string=w50:string)  [unwired: 1 in]
      n42 = Number To Decimal String(number=w49) -> (decimal integer string=w48:string)  [unwired: 1 in]
      n43 = Number To Fractional String(number=w47) -> (F-format string=w46:string)  [unwired: 3 in]
      n44 = Number To Decimal String(number=w45) -> (decimal integer string=w44:string)  [unwired: 1 in]
      n45 = Number To Decimal String(number=w21) -> (decimal integer string=w20:string)  [unwired: 1 in]
      n46 = Number To Fractional String(number=w19) -> (F-format string=w18:string)  [unwired: 3 in]
      n47 = Number To Decimal String(number=w17) -> (decimal integer string=w16:string)  [unwired: 1 in]
      n48 = Number To Decimal String(number=w162) -> (decimal integer string=w161:string)  [unwired: 1 in]
      n49 = Number To Decimal String(number=w160) -> (decimal integer string=w158:string)  [unwired: 1 in]
      n50 = Number To Decimal String(number=w157) -> (decimal integer string=w155:string)  [unwired: 1 in]
      n51 = Number To Decimal String(number=w142) -> (decimal integer string=w140:string)  [unwired: 1 in]
      n52 = Number To Decimal String(number=w139) -> (decimal integer string=w137:string)  [unwired: 1 in]
      n53 = Number To Decimal String(number=w125) -> (decimal integer string=w123:string)  [unwired: 1 in]
      n54 = Number To Decimal String(number=w122) -> (decimal integer string=w120:string)  [unwired: 1 in]
      n55 = Number To Decimal String(number=w119) -> (decimal integer string=w117:string)  [unwired: 1 in]
      n56 = Number To Decimal String(number=w116) -> (decimal integer string=w114:string)  [unwired: 1 in]
      n57 = Number To Decimal String(number=w113) -> (decimal integer string=w111:string)  [unwired: 1 in]
      n58 = Number To Decimal String(number=w105) -> (decimal integer string=w103:string)  [unwired: 1 in]
      n59 = Number To Decimal String(number=w102) -> (decimal integer string=w100:string)  [unwired: 1 in]
      n60 = Number To Decimal String(number=w96) -> (decimal integer string=w94:string)  [unwired: 1 in]
      n61 = Number To Fractional String(number=w90) -> (F-format string=w89:string)  [unwired: 3 in]
      n62 = Number To Fractional String(number=w88) -> (F-format string=w87:string)  [unwired: 3 in]
      n63 = Number To Fractional String(number=w86) -> (F-format string=w85:string)  [unwired: 3 in]
      n64 = Number To Fractional String(number=w84) -> (F-format string=w83:string)  [unwired: 3 in]
      n65 = Number To Fractional String(number=w82) -> (F-format string=w81:string)  [unwired: 3 in]
      n66 = Number To Fractional String(number=w80) -> (F-format string=w79:string)  [unwired: 3 in]
      n67 = Number To Decimal String(number=w78) -> (decimal integer string=w77:string)  [unwired: 1 in]
      n68 = Number To Decimal String(number=w76) -> (decimal integer string=w75:string)  [unwired: 1 in]
      n69 = Number To Decimal String(number=w74) -> (decimal integer string=w72:string)  [unwired: 1 in]
      n70 = Number To Fractional String(number=w71) -> (F-format string=w70:string)  [unwired: 3 in]
      n71 = Number To Fractional String(number=w69) -> (F-format string=w68:string)  [unwired: 3 in]
      n72 = Number To Fractional String(number=w67) -> (F-format string=w66:string)  [unwired: 3 in]
      n73 = Number To Decimal String(number=w65) -> (decimal integer string=w64:string)  [unwired: 1 in]
      n74 = Number To Decimal String(number=w42) -> (decimal integer string=w40:string)  [unwired: 1 in]
      n75 = Number To Decimal String(number=w39) -> (decimal integer string=w37:string)  [unwired: 1 in]
      n76 = Number To Decimal String(number=w36) -> (decimal integer string=w34:string)  [unwired: 1 in]
      n77 = Number To Decimal String(number=w30) -> (decimal integer string=w28:string)  [unwired: 1 in]
      n78 = Number To Decimal String(number=w27) -> (decimal integer string=w25:string)  [unwired: 1 in]
      n79 = Number To Decimal String(number=w24) -> (decimal integer string=w22:string)  [unwired: 1 in]
      n80 = Build Array(w176, w175, w174, w173, w172, w170, w169, w168, w167, w166, w164, w161, w158, w155, w154, w153, w152, w151, w150, w149, w148, w146, w144, w143, w140, w137, w135, w133, w131, w129, w127, w126, w123, w120, w117, w114, w111, w110, w109, w108, w106, w103, w100, w99, w97, w94, w93, w91, w89, w87, w85, w83, w81, w79, w77, w75, w72, w70, w68, w66, w64, w62, w60, w58, w56, w54, w52, w50, w48, w46, w44, w43, w40, w37, w34, w33, w32, w31, w28, w25, w22, w20, w18, w16, w15) -> (w14:string[])
    }
    frame "Dishwasher Kitchen" {
    }
    frame "HEWH", "PRAT", "HEWH RLT" {
      n81 = case shown="False" "Disable ERD (Main)" {
        tunnel: "HEWH ERD Data" -> [w191 _]
        tunnel: [w190 string[] []] -> w183
        frame False {
          n82 = case shown="False" FALSE {
            tunnel: w191 -> [w193 w252]
            tunnel: [w192 w199] -> w190
            frame False {
              n83 = Unbundle By Name(w193) -> ("ERD ENUM Data.User Set Point"=w196:dbl, "ERD ENUM Data.Actual Set Point"=w195:dbl, "Model Designator"=w197:u8, "ERD Therm Data.T6"=w194:dbl)
              n84 = Build Array(w196, w195, w197, w194) -> (w198:dbl[])
              n85 = call "UTILITY 1D DBL to 1D String.vi"("1D DBL"=w198) -> ("1D String"=w192:string[])  [unwired: 10 in]
            }
            frame True {
              n86 = Unbundle By Name(w252) -> ("ERD ENUM Data.User Set Point"=w251:dbl, "ERD ENUM Data.Vacation Set Point"=w250:dbl, "ERD ENUM Data.Actual Set Point"=w249:dbl, "ERD ENUM Data.Vacation Remaining\n6"=w248:dbl, "Model Designator"=w247:u8, "ERD Therm Data.T2"=w246:dbl, "ERD Therm Data.T3a"=w245:dbl, "ERD Therm Data.T3b"=w244:dbl, "ERD Therm Data.T4"=w243:dbl, "ERD Therm Data.T5"=w242:dbl, "ERD Therm Data.T6"=w241:dbl, "ERD Therm Data.Current"=w240:dbl, "ERD Therm Data.Voltage"=w237:dbl, "ERD Therm Data.EEV Possition"=w239:dbl, "ERD Therm Data.Actual Set Point"=w238:dbl, "ERD ENUM Data.Flow Events"=w264:string, "ERD ENUM Data.User Set Mode"=w263:string, "ERD ENUM Data.Operating Mode"=w262:string, "ERD ENUM Data.DRM Fallback Mode"=w261:string, "ERD ENUM Data.Vacation Fallback Mode"=w260:string, "ERD DRM Data.DRM Level"=w259:string, "ERD DRM Data.DRM Override"=w258:string, "ERD DRM Data.DRM Power"=w236:dbl, "ERD DRM Data.DRM Energy"=w235:dbl, "Fault Count.LE Fail"=w234:u32, "Fault Count.UE Fail"=w233:u32, "Fault Count.Comp Fail"=w232:u32, "Fault Count.Fan Fail"=w231:u32, "Fault Count.Dry Tank"=w230:u32, "Fault Count.Dirty Filter"=w229:u32, "Fault Count.T2 Fail"=w228:u32, "Fault Count.T3a Fail"=w227:u32, "Fault Count.T3b Fail"=w226:u32, "Fault Count.T4 Fail"=w225:u32, "Fault Count.T5 Fail"=w224:u32, "Fault Count.Cond A"=w223:u32, "Fault Count.Cond B"=w222:u32, "Fault Count.Cond C"=w221:u32, "Fault Count.Cond D"=w220:u32, "Fault Count.Cond E"=w219:u32, "Fault Count.Cond F"=w218:u32, "Fault Count.Cond G"=w217:u32, "Fault Count.Cond H"=w216:u32, "Fault Count.Cond I"=w215:u32, "Fault Count.Cond J"=w214:u32, "Fault Count.Cond L"=w213:u32, "Condensate Drain Pan Voltage"=w212:u16, "Relays.DLB"=w257:bool, "Relays.Comp"=w256:bool, "Relays.UE"=w255:bool, "Relays.LE"=w254:bool, "Relays.Fan"=w253:bool, "Comp Min On/Off Time"=w206:u16, "SS Run State"=w205:u16)
              n87 = Boolean To (0,1)(Boolean=w257) -> (0, 1=w211:i16)
              n88 = Boolean To (0,1)(Boolean=w256) -> (0, 1=w210:i16)
              n89 = Boolean To (0,1)(Boolean=w255) -> (0, 1=w209:i16)
              n90 = Boolean To (0,1)(Boolean=w254) -> (0, 1=w208:i16)
              n91 = Boolean To (0,1)(Boolean=w253) -> (0, 1=w207:i16)
              n92 = Build Array(w251, w250, w249, w248, w247, w246, w245, w244, w243, w242, w241, w240, w237, w239, w238) -> (w204:dbl[])
              n93 = Build Array(w264, w263, w262, w261, w260, w259, w258) -> (w201:string[])
              n94 = call "UTILITY 1D DBL to 1D String.vi"("1D DBL"=w204) -> ("1D String"=w202:string[])  [unwired: 10 in]
              n95 = Build Array(w236, w235, w234, w233, w232, w231, w230, w229, w228, w227, w226, w225, w224, w223, w222, w221, w220, w219, w218, w217, w216, w215, w214, w213, w212, w211, w210, w209, w208, w207, w206, w205) -> (w203:dbl[])
              n96 = call "UTILITY 1D DBL to 1D String.vi"("1D DBL"=w203) -> ("1D String"=w200:string[])  [unwired: 10 in]
              n97 = Build Array (concatenate)(w202, w201, w200) -> (w199:string[])
            }
          }
        }
        frame True {
        }
      }
      n98 = case shown="False" "Disable Electronic Mixing Valve (EMV) List" {
        tunnel: w183 -> [w282 w284]
        tunnel: [w282 w284] -> w186
        tunnel: "HEWH ERD Data" -> [w281 _]
        tunnel: [w266 string[] []] -> w184
        frame False {
          n99 = Unbundle By Name(w281) -> ("Mixing Valve.Tank Target Setpoint (0X4078)"=w280:dbl, "Mixing Valve.EMV Offset (0x4072)"=w279:dbl, "Mixing Valve.EMV Absolute Position (0x4073)"=w278:dbl, "Mixing Valve.Tank TCO State (0x4074)"=w271:string, "Mixing Valve.Outlet TCO State (0x4075)"=w270:string, "Mixing Valve.Fan PWM Drive %  (0x4076)"=w276:dbl, "Mixing Valve.T7 (0x407D)"=w275:dbl, "Mixing Valve.Cold Water Supply Temperature (0x40B7)"=w274:dbl, "Mixing Valve.Mixing Valve Flow State (0x407E)"=w268:string, "Mixing Valve.Mixing Valve PID Override (0x407F)"=w267:string)
          n100 = Build Array(w280, w279, w278) -> (w277:dbl[])
          n101 = Build Array(w276, w275, w274) -> (w273:dbl[])
          n102 = call "UTILITY 1D DBL to 1D String.vi"("1D DBL"=w277) -> ("1D String"=w272:string[])  [unwired: 10 in]
          n103 = call "UTILITY 1D DBL to 1D String.vi"("1D DBL"=w273) -> ("1D String"=w269:string[])  [unwired: 10 in]
          n104 = Build Array (concatenate)(w272, w271, w270, w269, w268, w267) -> (w266:string[])
        }
        frame True {
        }
      }
      n105 = Build Array (concatenate)(w186, w184) -> (w182:string[])
    }
    frame "Dryer" {
    }
  }
  "Error Out" <- w7
  n106 = disable-structure shown="Disabled" {
    frame Disabled {
      (unwired) string[] ["Critical Major (0x0100)", "Critical Minor (0x0100)", "Non-Critical Major (0x0100)", "Non-Critical Minor (0x0100)", "Daily Revision (0x0100)", "Cycle Count (0x2003)", "XML Critical Major (0xF001)", "XML Critical Minor (0xF001)", "XML Non-Critical Major (0xF001)", "XML Non-Critical Minor (0xF001)", "Available Free Stack % (0xF014)", "Extra Rinse (0xF101)", "Deep Rinse_Fabric Softener (0xF102)", "My Cycle (0xF103)", "Soil Level (0xF105)", "Spin Level (0xF106)", "Stain (0xF107)", "Temperature Level (0xF108)", "Load Size (0xF109)", "Machine State (0xF10A)", "Cycle Selected (0xF10C)", "Delay Time (0xF10D)", "Soak Time (0xF10E)", "Auto Soak Level (0xF11E)", "Deep Fill (0xF123)", "Warm Rinse (0xF124)", "Remaining Cycle Time(s) (0xF140)", "Wet Load Gallons (0xF200)", "Tub Volume Gallons (0xF201)", "Pressure (inches of H20) (0xF202)", "Target Gallons (0xF205)", "Load Type (0xF206)", "Lid Switch (0xF207)", "Hot Water Valve (0xF209)", "Cold Water Valve (0xF209)", "Spray_Rinse Valve (0xF209)", "Fabric Softener Valve (0xF209)", "Lid Lock Req State (0xF20A)", "Lid Lock Status (0xF20B)", "Cycle Engine State (0xF20C)", "Current Water Temperature (°F) (0xF20F)", "Drain Pump (0xF210)", "Recirculating Pump (0xF211)", "Sub-Cycle (0xF213)", "Target Level Inches (0xF215)", "Valve Relay (0xF218)", "Lid Lock FB (0xF219)", "Target Bath Temperature (°F) (0xF221)", "Current Bath Temperature (°F) (0xF222)", "Cold Inlet Temperature (°F) (0xF223)", "Hot Inlet Temperature (°F) (0xF224)", "Warm Inlet Temperature (°F) (0xF225)", "Hot Gallons (0xF226)", "Cold Gallons (0xF226)", "Hot Seg Valve Time (0xF227)", "Cold Seg Valve Time (0xF227)", "Child Safety (0xF22A)", "Segment Gallons (0xF22B)", "Ramp Average Current (0xF300)", "Coast Line Voltage (0xF301)", "Ramp Speed (0xF302)", "Ramp Time (0xF303)", "Coast Time (0xF304)", "Dry Load Size (0xF305)", "Folding in Acceleration (0xF306)", "Max Jerk In Acceleration (0xF307)", "Max Jerk In S-S (0xF308)", "Shaft Speed (RPM) (0xF30A)", "Basket Speed (RPM) (0xF30B)", "Current RMS (Amps) (0xF30D)", "Target Speed (RPM) (0xF30E)", "Motor Mode (0xF313", "OOB Detected in Acceleration (0xF315)", "OOB Detected in S-S (0xF316)", "OOB ReDistribution Required (0xF317)", "Motor Profile Status (0xF319)", "Motor Profile (0xF319)", "Mode Shift Status (0xF31D)", "ME Relay (0xF321)", "Mode Shift FB (0xF322)", "MS Motor (0xF323)", "Partial Coast Time (0xF32D)", "Ramp Line Voltage (0xF32E)", "Personality (0xF000)", "Reset Source (0xF017)"]
      (unwired) string[] ["TANKSETPOINT (0X4078)", "MIXVALVESTEPOFFSET (0x4072)", "MIXVALVESTEPABSOLUTE (0x4073)", "FIRSTSTAGEKPGAIN (0x4074)", "FIRSTSTAGEKIGAIN (0x4075)", "FIRSTSTAGEKDGAIN (0X4076)", "FIRSTSTAGEKPQBITS (0x4079)", "FIRSTSTAGEKIQBITS (0x407A)", "FIRSTSTAGEKDQBITS (0x407B)", "SECONDSTAGEKPGAIN (0x408E)", "SECONDSTAGEKIGAIN (0x408F)", "SECONDSTAGEKDGAIN (0x4090)", "SECONDSTAGEKPQBITS (0x4091)", "SECONDSTAGEKIQBITS (0x4092)", "SECONDSTAGEKDQBITS (0x4093)", "THIRDSTAGEKPGAIN (0x4094)", "THIRDSTAGEKIGAIN (0x4095)", "THIRDSTAGEKDGAIN (0x4096)", "THIRDSTAGEKPQBITS (0x4097)", "THIRDSTAGEKIQBITS (0x4098)", "THIRDSTAGEKDQBITS (0x4099)", "FOURTHSTAGEKPGAIN (0x409A)", "FOURTHSTAGEKIGAIN (0x409B)", "FOURTHSTAGEKDGAIN (0x409C)", "FOURTHSTAGEKPQBITS (0x409D)", "FOURTHSTAGEKIQBITS (0x409E)", "FOURTHSTAGEKDQBITS (0x409F)", "MIXVALVEDELTAT (0x4077)", "PIDOUTPUTPOSITION (0x407C)"]
      (unwired) string[] ["USERSETPOINT (0x4024)", "VACATIONSETPOINT (0x4025)", "ACTUALSETPOINT (0x4026)", "TIMEDHOURSREMAINING (0x4028)", "MODELDESIGNATOR (0x4042)", "T2TEMP (0x4060)", "T3ATEMP (0x4061)", "T3BTEMP (0x4062)", "T4TEMP (0x4063)", "T5TEMP (0x4064)", "T6TEMP (0x406E)", "Current (0x4065)", "Voltage (0x4066)", "EEV Position (0x4067)", "Actual Set Point (0x4026)", "Flow Events (0x4069)", "User Set Mode (0x4020)", "Operating Mode (0x4021)", "DRM Fallback (0x4022)", "Vacation Fallback (0x4023)", "DRM Level (0xD000)", "DRM Override State (0xD001)", "DRM Power (0xD007)", "DRM Energy (0xD008)", "Fault Counts - LE Fail (0x4045)", "Fault Counts - UE Fail (0x4045)", "Fault Counts - Compressor Fail (0x4045)", "Fault Counts - Fan Fail (0x4045)", "Fault Counts - Dry Tank (0x4045)", "Fault Counts - Dirty Filter (0x4045)", "Fault Counts - T2 Fail (0x4045)", "Fault Counts - T3a Fail (0x4045)", "Fault Counts - T3b Fail (0x4045)", "Fault Counts - T4 Fail (0x4045)", "Fault Counts - T5 Fail (0x4045)", "Fault Counts - Cond A (0x4045)", "Fault Counts - Cond B (0x4045)", "Fault Counts - Cond C (0x4045)", "Fault Counts - Cond D (0x4045)", "Fault Counts - Cond E (0x4045)", "Fault Counts - Cond F (0x4045)", "Fault Counts - Cond G (0x4045)", "Fault Counts - Cond H (0x4045)", "Fault Counts - Cond I (0x4045)", "Fault Counts - Cond J (0x4045)", "Fault Counts - Cond L (0x4045)", "Condensor Drain Pan Voltage (0x4071)", "Relay States - DLB (0x4068)", "Relay States - Compressor (0x4068)", "Relay States - Upper Element (0x4068)", "Relay States - Lower Element (0x4068)", "Relay States - Fan (0x4068)", "Compressor Min On/Off Time (0x406B)", "SS Run State (0x406C)"]
    }
    frame Enabled {
    }
  }
  n107 = for {
    tunnel: "Headers" -> [w289] mode=indexing
    tunnel: [w288] -> w5 mode=indexing
    w287 = T12 0 items=["both", "start of string", "end of string"] ("location (both)")
    n108 = call <vilib>:"Trim Whitespace.vi"("string"=w289, "location (both)"=w287) -> ("trimmed string"=w288:string)
  }
  n109 = for {
    tunnel: w2 -> [w292] mode=indexing
    tunnel: [w291] -> w1 mode=indexing
    w290 = T12 0 items=["both", "start of string", "end of string"] ("location (both)")
    n110 = call <vilib>:"Trim Whitespace.vi"("string"=w292, "location (both)"=w290) -> ("trimmed string"=w291:string)
  }
  n111 = for {
    tunnel: "Raw Data" -> [w295] mode=indexing
    tunnel: [w294] -> w3 mode=indexing
    w293 = T12 0 items=["both", "start of string", "end of string"] ("location (both)")
    n112 = call <vilib>:"Trim Whitespace.vi"("string"=w295, "location (both)"=w293) -> ("trimmed string"=w294:string)
  }
  n113 = Build Array(w5, w1, w3) -> (w11:string[][])
  n114 = Transpose 2D Array(2D array=w11) -> (transposed array=→"ERD Array":string[][])
